vi "create node queue refnum.vi"(8 "error in":errorcluster, 11 "Subscriber name":string) -> (0 "error out":errorcluster, 3 "queue out":refnum<queue>)   [LabVIEW 2023, in "Publisher Subscriber.lvlib"]
uses:
  <userlib>/_Publisher Subscriber/Publisher Subscriber.lvlib
  <userlib>/_Publisher Subscriber/Controls/data cluster.ctl
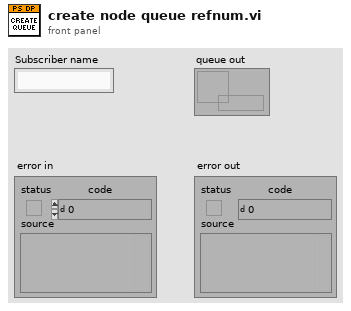
[diagram p1: front panel]
types:
  T1 = typedef "Publisher Subscriber.lvlib/data cluster.ctl" = cluster{"Command":string, "Data":variant}
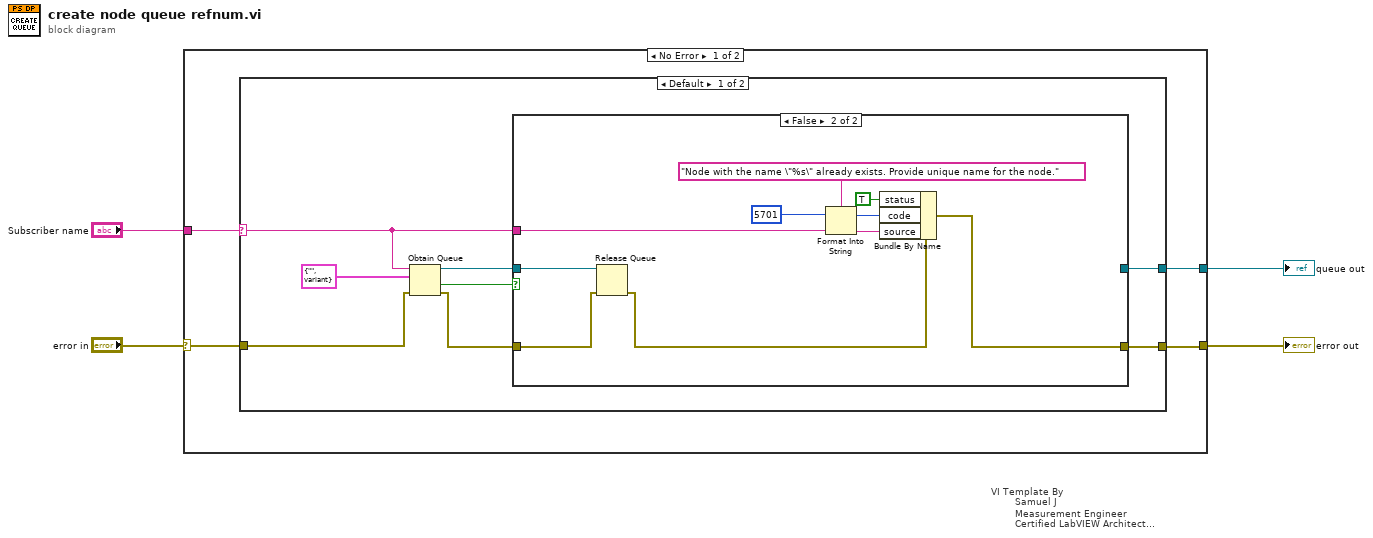
[diagram p0: block diagram]
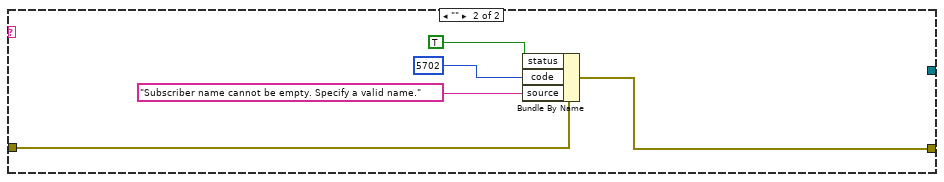
[diagram p3: hidden frame]
diagram:
  n1 = case "VI Template By\n        Samuel J\n        Measurement Engineer\n        Certified LabVIEW Architect\n        Vestas Technology R&D Chennai" shown="No Error" "error in" {
    selector: "error in" -> [w8 w33]
    tunnel: [w7 w33] -> w3
    tunnel: "Subscriber name" -> [w6 _]
    tunnel: [w5 _] -> w1
    frame No Error {
      n2 = case shown="Default" w6 {
        selector: w6 -> [w11 _]
        tunnel: w8 -> [w15 w30]
        tunnel: [w14 w29] -> w7
        tunnel: [w10 _] -> w5
        frame Default {
          n3 = Obtain Queue(name (unnamed)=w11, element data type=T1 {"Command"="", "Data"=variant} ("Data Cluster"), error in (no error)=w15) -> (queue out=w9:refnum<queue>, created new?=w12:bool, error out=w13:errorcluster)  [unwired: 2 in]
          n4 = case shown="False" w12 {
            tunnel: [w18 w27] -> w14
            tunnel: w13 -> [w18 w19]
            tunnel: w11 -> [_ w22]
            tunnel: [w17 _] -> w10
            tunnel: w9 -> [w17 w21]
            frame True {
            }
            frame False {
              n5 = Release Queue(queue=w21, error in (no error)=w19) -> (error out=w20:errorcluster)  [unwired: 1 in, 2 out]
              n6 = Format Into String(format string="Node with the name \"%s\" already exists. Provide unique name for the node." ("source"), w22) -> (resulting string=w25:string)  [unwired: 2 in, 1 out]
              n7 = Bundle By Name(cluster=w20, "status"=TRUE, "code"=5701, "source"=w25) -> (w27:errorcluster)
            }
          }
        }
        frame "" {
          n8 = Bundle By Name(cluster=w30, "status"=TRUE, "code"=5702, "source"="Subscriber name cannot be empty. Specify a valid name.") -> (w29:errorcluster)
        }
      }
    }
    frame Error {
    }
  }
  "error out" <- w3
  "queue out" <- w1
